vi "5181_RF_Off.vi"(2 "error in (no error)":errorcluster, 3 "address":string) -> (0 "error out":errorcluster, 1 "address out":string)   [LabVIEW 2013]
doc: "This device configures the Rohde & Schwarz RF Generator for use. The central frequency, modulation, RF power, and GPIB address are taken from the QCA Global."
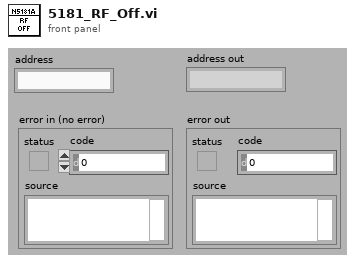
[diagram p1: front panel]
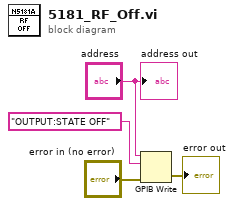
[diagram p0: block diagram]
diagram:
  n1 = GPIB Write(0:"address", 1:"OUTPUT:STATE OFF", 3:"error in (no error)") -> (6:→"error out":errorcluster)  [unwired: 2 in, 1 out]
  "address out" <- "address"
